vi "update status.vi"(8 "error in (no error)":errorcluster, 10 "status in":string, 11 "Thorcam in":refnum<class "Thorcam.lvclass">) -> (0 "error out":errorcluster, 3 "Thorcam out":refnum<class "Thorcam.lvclass">)   [LabVIEW 2012, in "Thorcam.lvclass"]
uses:
  Thorcam.lvclass
  Thorcam.lvclass/Thorcam.ctl
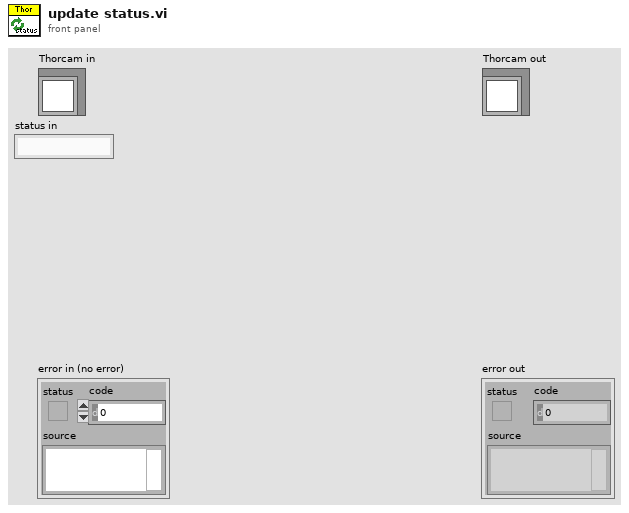
[diagram p1: front panel]
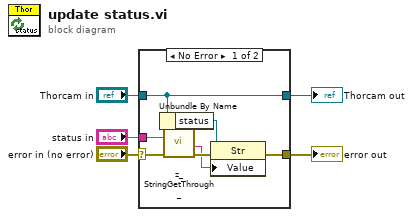
[diagram p0: block diagram]
diagram:
  n1 = case shown="No Error" "error in (no error)" {
    selector: "error in (no error)" -> [w11 w14]
    tunnel: [w8 w14] -> w4
    tunnel: [w12 w13] -> w2
    tunnel: "Thorcam in" -> [w12 w13]
    tunnel: "status in" -> [w10 _]
    frame No Error {
      n2 = Unbundle By Name(w12) -> ("status"=w7:refnum<vi>)
      n3 = call <instrlib>:"z_StringGetThrough_.vi"("Error In"=w11, "String In"=w10) -> ("Error Out"=w9:errorcluster, "String Out"=w6:string)  [unwired: 8 in]
      n4 = property class="Str"(reference=w7, error in=w9, "Value"=w6) -> (error out=w8:errorcluster)  [unwired: 1 out]
    }
    frame Error {
    }
  }
  "error out" <- w4
  "Thorcam out" <- w2
